vi "connect4g_v0.vi"() -> ()   [LabVIEW 2016]
panel:
  out "own_IP":string
  out "data size [byte]":i32
  out "incoming data":bool
  out "TCP":errorcluster
  out "server connected":bool
  in  "broadcast_port":u16=9000
  in  "send_to_IP":string="127.0.0.1"
  out "udp":errorcluster
  in  "stop":bool
  out "Tried to connect":i32
  in  "server_port":u16=9999
  in  "server_IP":string="5.38.239.10"
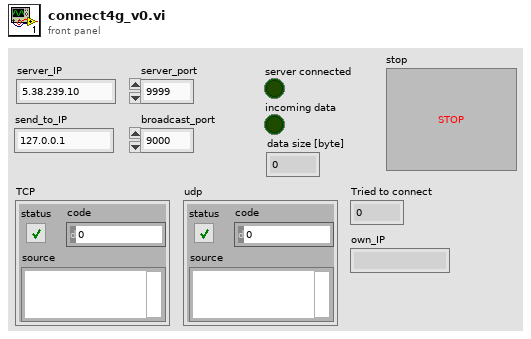
[diagram p1: front panel]
types:
  T1 = enum16{"Standard", "Buffered", "CRLF", "Immediate"}
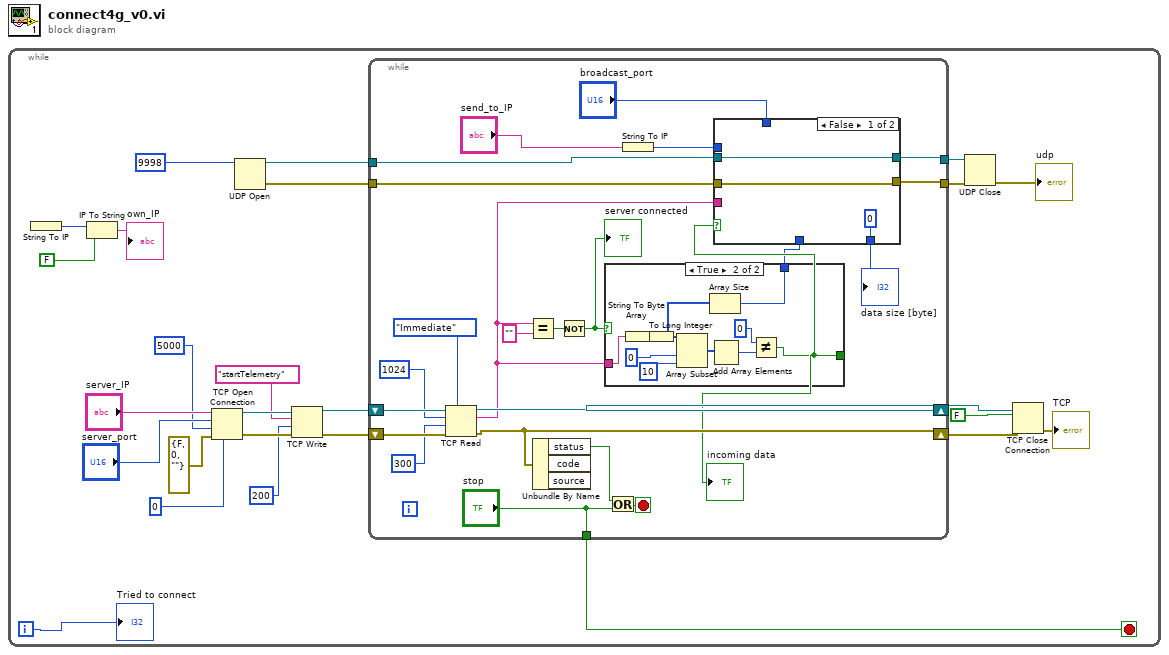
[diagram p0: block diagram]
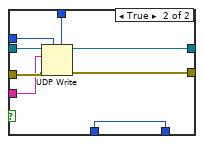
[diagram p2: hidden frame]
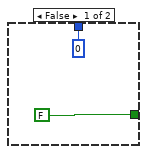
[diagram p3: hidden frame]
diagram:
  n1 = while {
    i -> [w8]
    stop <- w6 stop-if-true
    n2 = String To IP() -> (0:w3:u32)  [unwired: 1 in]
    n3 = IP To String(1:FALSE ("dot notation? (F)"), 2:w3) -> (0:→"own_IP":string)
    n4 = TCP Open Connection(address="server_IP", remote port or service name="server_port", timeout ms (60000)=5000, local port=u16 0 ("local port (0)"), error in (no error)=errorcluster {"status"=FALSE, "code"=0, "source"=""}) -> (connection ID=w23:refnum<k5>, error out=w22:errorcluster)
    n5 = UDP Open(11:u16 9998 ("port")) -> (port=w13:refnum<k16>, 0:w14:errorcluster)  [unwired: 4 in, 1 out]
    n6 = TCP Write(connection ID=w23, data in="startTelemetry", error in (no error)=w22, 9:200 ("timeout ms (25000)")) -> (connection ID out=w19:refnum<k5>, error out=w18:errorcluster)  [unwired: 1 out]
    n7 = while {
      shift-right: [w48] -> w17
      shift-left: w19 -> [w50]
      shift-right: [w43] -> w9
      shift-left: w18 -> [w49]
      tunnel: [w37] -> w15
      tunnel: w14 -> [w36]
      tunnel: w13 -> [w35]
      tunnel: [w34] -> w12
      tunnel: ["stop"] -> w6
      stop <- w44 stop-if-true
      n8 = TCP Read(connection ID=w50, bytes to read=1024, error in (no error)=w49, 7:T1."Immediate" ("mode (standard)"), 9:300 ("timeout ms (25000)")) -> (connection ID out=w48:refnum<k5>, data out=w33:string, error out=w43:errorcluster)
      n9 = Equal?(x=w33, y="") -> (x = y?=w39:bool)
      n10 = Unbundle By Name(w43) -> ("status"=w41:bool)  [unwired: 2 out]
      n11 = Not(x=w39) -> (.not. x?=w38:bool)
      "server connected" <- w38
      n12 = case shown="True" w38 {
        tunnel: w33 -> [_ w73]
        tunnel: [FALSE w66] -> w32
        tunnel: [0 w64] -> w28
        frame False {
        }
        frame True {
          n13 = String To Byte Array(string=w73) -> (unsigned byte array=w72:u8[])
          n14 = To Long Integer(number=w72) -> (32bit integer=w65:i32[])
          n15 = Array Subset(array=w65, index=0, length=10) -> (w69:i32[])
          n16 = Array Size(array=w65) -> (size(s)=w64:i32)
          n17 = Add Array Elements(numeric array=w69) -> (sum=w68:i32)
          n18 = Not Equal?(x=0, y=w68) -> (x != y?=w66:bool)
        }
      }
      "incoming data" <- w32
      n19 = Or(x=w41, y="stop") -> (x .or. y?=w44:bool)
      n20 = String To IP(1:"send_to_IP") -> (0:w31:u32)
      n21 = case shown="False" w32 {
        tunnel: [w52 w61] -> w37
        tunnel: w36 -> [w52 w60]
        tunnel: w35 -> [w53 w59]
        tunnel: [w53 w58] -> w34
        tunnel: w33 -> [_ w57]
        tunnel: w31 -> [_ w56]
        tunnel: "broadcast_port" -> [_ w55]
        tunnel: w28 -> [_ w54]
        tunnel: [0 w54] -> w27
        frame False {
        }
        frame True {
          n22 = UDP Write(address=w56, port or service name=w55, connection ID=w59, data in=w57, 8:w60) -> (error out=w61:errorcluster, 3:w58:refnum<k16>)  [unwired: 1 in]
        }
      }
      "data size [byte]" <- w27
    }
    n23 = UDP Close(connection ID=w12, 8:w15) -> (error out=→"udp":errorcluster)  [unwired: 1 out]
    n24 = TCP Close Connection(connection ID=w17, abort (F)=FALSE, error in (no error)=w9) -> (error out=→"TCP":errorcluster)  [unwired: 1 out]
    "Tried to connect" <- w8
  }
